vi "MGCC_FntStaMach_subMG_Identification.vi"(6 "Abnormal_enable_input":bool[][](array[boolean]), 7 "Abnormal input":string[](array[string]), 9 "Previous_states 2":string[](array[string]), 10 "Previous_node":i32[](array[numeric]), 11 "Turns":dbl) -> (0 "error out 2":errorcluster, 1 "Next_States":string[](array[string]), 3 "Next_node":dbl[](array[numeric]), 4 "Abnormal_enable_output":bool[][](array[boolean]), 5 "Abnormal_output":string[](array[string]))   [LabVIEW 2016]
uses:
  <vilib>/imath/engines/lvmath/Plug In/_Char/NIMS_CH_character datatype.ctl
  MGCC_FntStaMach_gobal.vi
  <vilib>/Utility/error.llb/Error Cluster From Error Code.vi
  <vilib>/imath/engines/lvmath/Plug In/_Char/NIMS_CH_String to Character Array.vi
  <vilib>/imath/engines/lvmath2/RunTimeEngine/RunTimeType/NIMS_RunTimeType_From StrictType (excl LVString).vi
  <instcachedir>/0/NIMS_RunTimeType_From StrictType (excl LVString)_BBF44FB49F834B71AF7A14CCEDF8BECD.lvgen/NIMS_RunTimeType_From StrictType (excl LVString)_BBF44FB49F834B71AF7A14CCEDF8BECD_006.vi
  <vilib>/imath/engines/lvmath2/RunTimeEngine/Struct/NIMS_StructSetField.vi
  <vilib>/imath/engines/lvmath2/RunTimeEngine/IndexRead/NIMS M(S,$).vi
  <instcachedir>/0/NIMS M(S,$)_F24F360562DE41D8BE234322A2E15C65.lvgen/NIMS M(S,$)_F24F360562DE41D8BE234322A2E15C65_000.vi
  <vilib>/imath/engines/lvmath2/RunTimeEngine/BuiltInFunctions/findnz/NIMS_[1o]_findnz(GRowV).vi
  <instcachedir>/0/NIMS_[1o]_findnz(GRowV)_1AF74843B4874134ADE908C0A4A72F3C.lvgen/NIMS_[1o]_findnz(GRowV)_1AF74843B4874134ADE908C0A4A72F3C_000.vi
  <vilib>/imathl/engines/lvmath/Functions/Error Handling/Create Error.vi
  <vilib>/imath/engines/lvmath2/RunTimeEngine/BuiltInFunctions/length/NIMS_length(GV).vi
  <instcachedir>/0/NIMS_length(GV)_08A3D13377FD4E4B96F5795FBF3698FA.lvgen/NIMS_length(GV)_08A3D13377FD4E4B96F5795FBF3698FA_000.vi
  <vilib>/imath/engines/lvmath2/RunTimeEngine/RangeToken/NIMS_Range_R3 - Integer.vi
  <instcachedir>/0/NIMS_Range_R3 - Integer_A435E2FF893B4C718FD5055FE39FE2F6.lvgen/NIMS_Range_R3 - Integer_A435E2FF893B4C718FD5055FE39FE2F6_000.vi
  <vilib>/imath/engines/lvmath2/RunTimeEngine/CommandStatement/MC_CommandStatement_break.vi
  <vilib>/imath/engines/lvmath2/RunTimeEngine/BuiltInFunctions/is_empty/NIMS_is_empty(GV).vi
  <instcachedir>/0/NIMS_is_empty(GV)_FC7E7C3D9544432CB6AA2416ADCF6D56.lvgen/NIMS_is_empty(GV)_FC7E7C3D9544432CB6AA2416ADCF6D56_000.vi
  <vilib>/imath/engines/lvmath2/RunTimeEngine/IndexRead/NIMS M($,S).vi
  <instcachedir>/0/NIMS M($,S)_3E5749BBB62E49528D4765A77F1F6D98.lvgen/NIMS M($,S)_3E5749BBB62E49528D4765A77F1F6D98_000.vi
  <vilib>/imath/engines/lvmath2/RunTimeEngine/RowToken/NIMS_RowToken_M_CV.vi
  <instcachedir>/0/NIMS_RowToken_M_CV_FA79F1D1D17D44459F3ED8E09EE8B625.lvgen/NIMS_RowToken_M_CV_FA79F1D1D17D44459F3ED8E09EE8B625_000.vi
  <vilib>/imath/engines/lvmath2/RunTimeEngine/ErrorHandling/NIMS_Create Error From Enums.vi
  <vilib>/imath/engines/lvmath2/RunTimeEngine/IndexRead/NIMS V(S).vi
  <instcachedir>/0/NIMS V(S)_0488751826AF41519A22953C041130DC.lvgen/NIMS V(S)_0488751826AF41519A22953C041130DC_000.vi
  <vilib>/imath/engines/lvmath2/RunTimeEngine/IndexRead/NIMS V(V).vi
  <instcachedir>/0/NIMS V(V)_298D9CB7BFEB42B8BC8D9C3C28AE8C70.lvgen/NIMS V(V)_298D9CB7BFEB42B8BC8D9C3C28AE8C70_002.vi
  <vilib>/imath/engines/lvmath2/RunTimeEngine/IndexReplace/NIMS V(S)=V.vi
  <instcachedir>/0/NIMS V(S)=V_623363232DF04CF88CEE4AC156064DF2.lvgen/NIMS V(S)=V_623363232DF04CF88CEE4AC156064DF2_003.vi
  <instcachedir>/0/NIMS_[1o]_findnz(GRowV)_1AF74843B4874134ADE908C0A4A72F3C.lvgen/NIMS_[1o]_findnz(GRowV)_1AF74843B4874134ADE908C0A4A72F3C_002.vi
  <vilib>/imath/engines/lvmath2/RunTimeEngine/VariableToken/NIMS_VariableToken_CondDefinedDefinedByReplace.vi
  <instcachedir>/0/NIMS_VariableToken_CondDefinedDefinedByReplace_D162CFFC24174562A9FEA619A91E1A56.lvgen/NIMS_VariableToken_CondDefinedDefinedByReplace_D162CFFC24174562A9FEA619A91E1A56_006.vi
  <vilib>/imath/engines/lvmath2/RunTimeEngine/IndexReplace/NIMS V(S)=S.vi
  <instcachedir>/0/NIMS V(S)=S_57E16554CB8B4B90AAB163894F717546.lvgen/NIMS V(S)=S_57E16554CB8B4B90AAB163894F717546_002.vi
  <vilib>/imath/engines/lvmath2/RunTimeEngine/BuiltInFunctions/size/NIMS_[I32,I32]=size(GM).vi
  <instcachedir>/0/NIMS_[I32,I32]=size(GM)_B0A6EC1255BB4C8AB801FE6F734128D9.lvgen/NIMS_[I32,I32]=size(GM)_B0A6EC1255BB4C8AB801FE6F734128D9_000.vi
  <vilib>/imath/engines/lvmath2/RunTimeEngine/Struct/NIMS_Struct_Cell Array To String Array.vi
  <vilib>/imath/engines/lvmath2/RunTimeEngine/IndexRead/NIMS V(R2).vi
  <instcachedir>/0/NIMS V(R2)_C76619605A0E4E9F8B2FA9389712AC47.lvgen/NIMS V(R2)_C76619605A0E4E9F8B2FA9389712AC47_002.vi
  <vilib>/imath/engines/lvmath2/RunTimeEngine/NodeEndStatement/NIMS_NodeEndStatement_Output.vi
  <instcachedir>/0/NIMS_NodeEndStatement_Output_53EC0D466D134D7ABD903AC30B43404B.lvgen/NIMS_NodeEndStatement_Output_53EC0D466D134D7ABD903AC30B43404B_004.vi
  <instcachedir>/0/NIMS_NodeEndStatement_Output_53EC0D466D134D7ABD903AC30B43404B.lvgen/NIMS_NodeEndStatement_Output_53EC0D466D134D7ABD903AC30B43404B_002.vi
  <instcachedir>/0/NIMS_NodeEndStatement_Output_53EC0D466D134D7ABD903AC30B43404B.lvgen/NIMS_NodeEndStatement_Output_53EC0D466D134D7ABD903AC30B43404B_031.vi
  <instcachedir>/0/NIMS_NodeEndStatement_Output_53EC0D466D134D7ABD903AC30B43404B.lvgen/NIMS_NodeEndStatement_Output_53EC0D466D134D7ABD903AC30B43404B_005.vi
  <vilib>/imath/engines/lvmath2/RunTimeEngine/ErrorHandling/NIMS_Finalize Error.vi
  <vilib>/ErrorRing/Error Ring.xnode
panel:
  out "emptyarray":i32[](array[numeric])
  out "temp_node":dbl[][](array[numeric])
  out "Next_states":string[](array[string])
  out "error out":errorcluster
  out "f_MGCC_OnliTopolden_node":dbl[][](array[numeric])
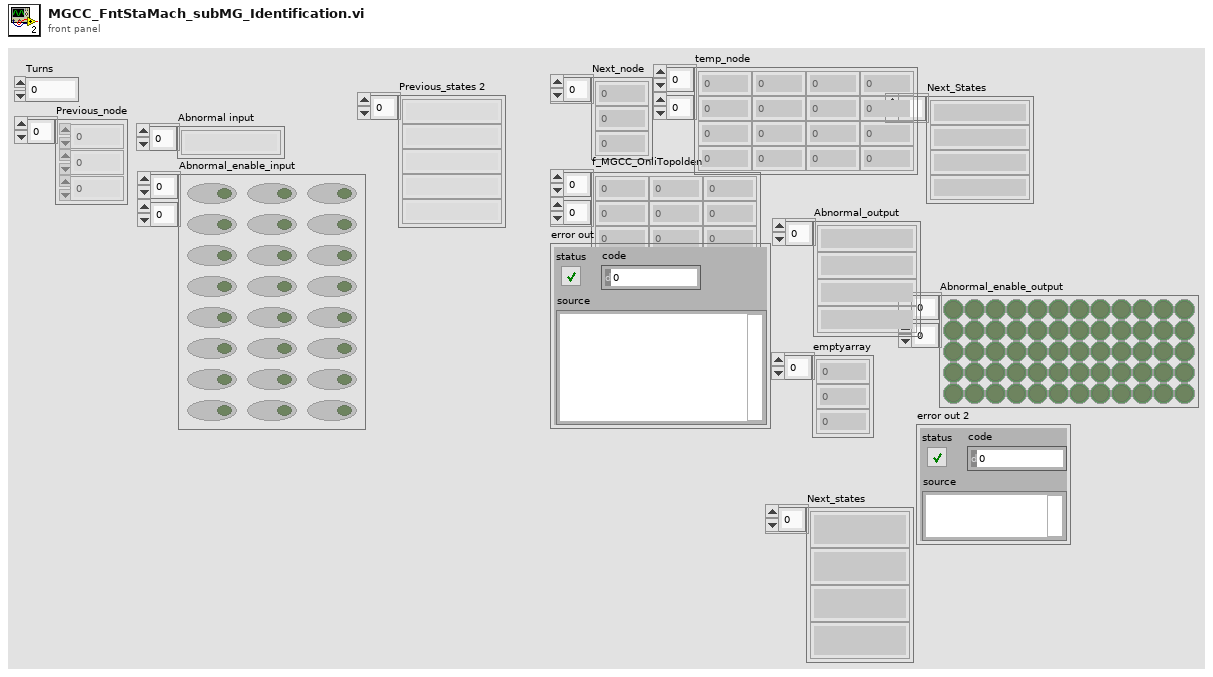
[diagram p1: front panel]
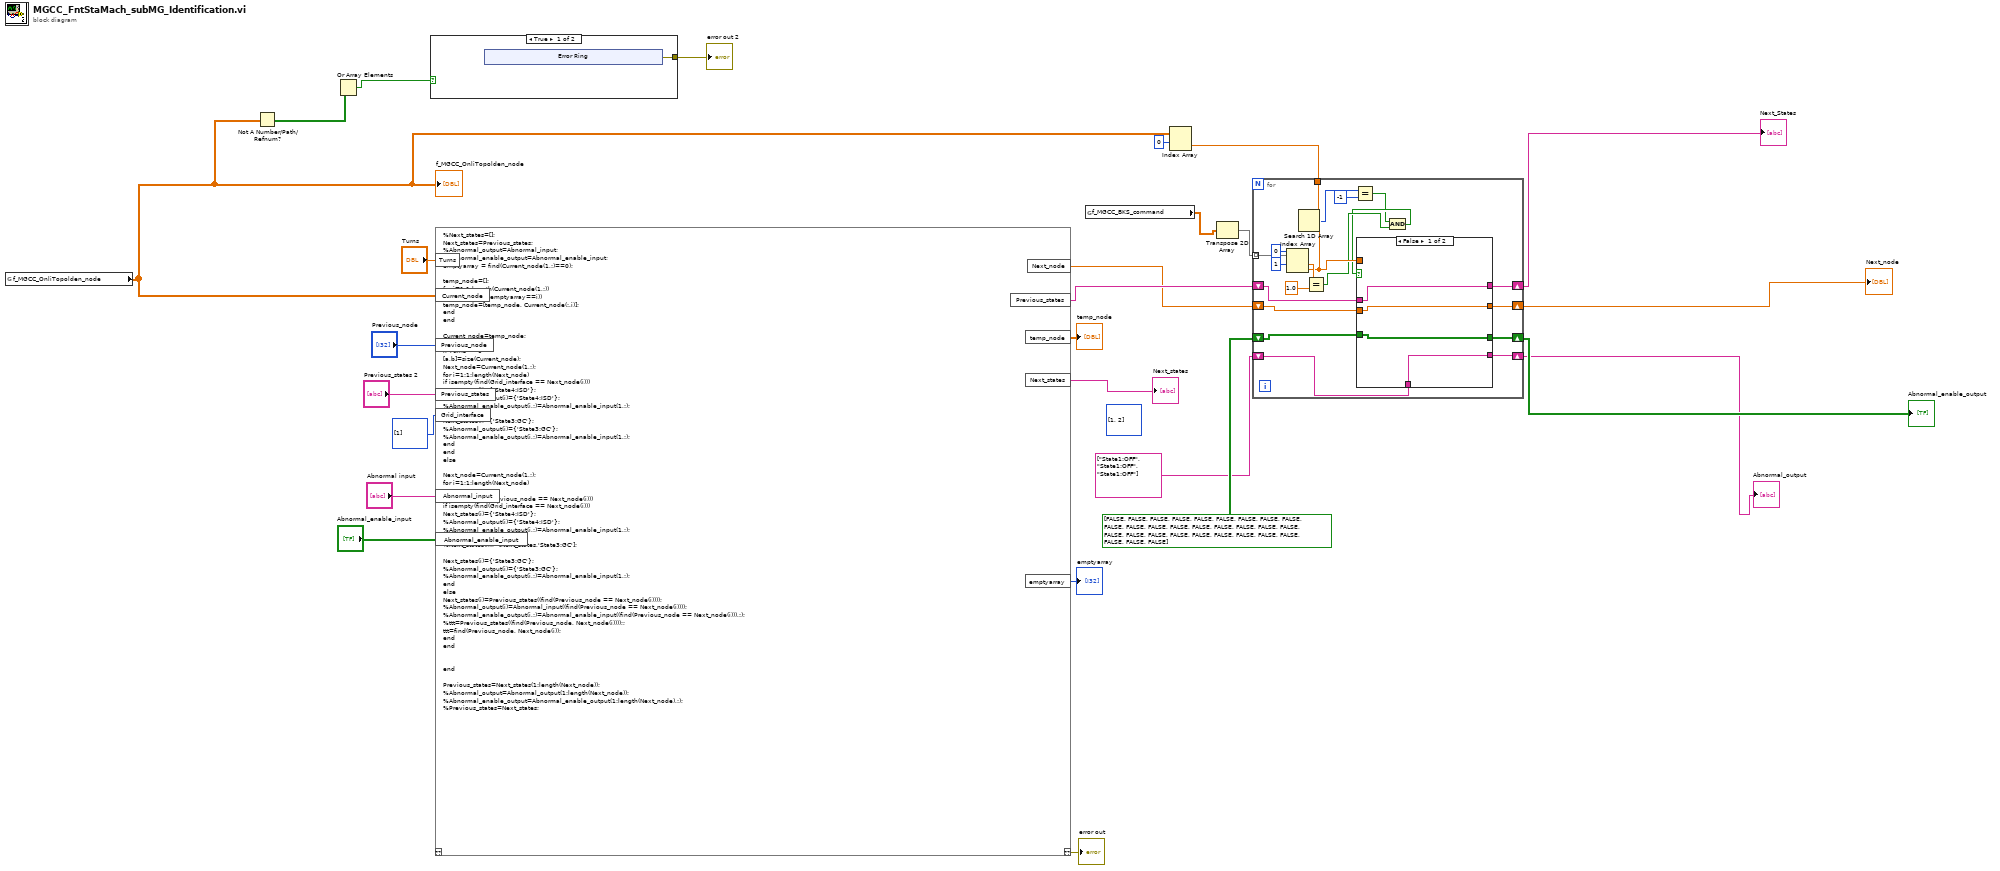
[diagram p0: block diagram]
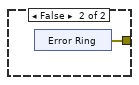
[diagram p2: hidden frame]
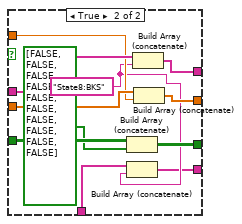
[diagram p3: hidden frame]
diagram:
  (unwired) i32[] [1, 2]
  n1 = global read "MGCC_FntStaMach_gobal.vi" "f_MGCC_OnliTopolden_node"() -> (w3:dbl[][])
  "f_MGCC_OnliTopolden_node" <- w3
  n2 = Not A Number/Path/Refnum?(number/path/refnum=w3) -> (NaN/Path/Refnum?=w8:bool[][])
  n3 = Or Array Elements(Boolean array=w8) -> (logical OR=w7:bool)
  n4 = case shown="True" w7 {
    tunnel: [w27 w33] -> w6
    frame True {
      n5 = xnode "Error Ring"() -> ("error out"=w27:errorcluster)
    }
    frame False {
      n6 = xnode "Error Ring"() -> ("error out"=w33:errorcluster)
    }
  }
  "error out 2" <- w6
  n7 = mathscript code="%Next_states=[];\nNext_states=Previous_states;\n%Abnormal_output=Abnormal_input;\n%Abnormal_enable_output=Abnormal_enable_input;\nemptyarray = find(Current_node(1,:)==0);\n\ntemp_node=[];\nfor i=1:1:length(Current_node(1,:))\nif isempty(find(emptyarray==i))\ntemp_node=[temp_node, Current_node(:,i)];\nend\nend\n\nCurrent_node=temp_node;\n\nif Turns ==0\n[a,b]=size(Current_node);\nNext_node=Current_node(1,:);\nfor i=1:1:length(Next_node)\nif isempty(find(Grid_interface == Next_node(i)))\nNext_states(i)={'State4:ISD'};\n%Abnormal_output(i)={'State4:ISD'};\n%Abnormal_enable_output(i,:)=Abnormal_enable_input(1,:);\nelse\nNext_states(i)={'State3:GC'};\n%Abnormal_output(i)={'State3:GC'};\n%Abnormal_enable_output(i,:)=Abnormal_enable_input(1,:);\nend\nend\nelse\n\nNext_node=Current_node(1,:);\nfor i=1:1:length(Next_node)\n\nif isempty(find(Previous_node == Next_node(i)))\nif isempty(find(Grid_interface == Next_node(i)))\nNext_states(i)={'State4:ISD'};\n%Abnormal_output(i)={'State4:ISD'};\n%Abnormal_enable_output(i,:)=Abnormal_enable_input(1,:);\nelse\n%Next_states(i,:)=[Next_states,'State3:GC'];\n\nNext_states(i)={'State3:GC'};\n%Abnormal_output(i)={'State3:GC'};\n%Abnormal_enable_output(i,:)=Abnormal_enable_input(1,:);\nend\nelse\nNext_states(i)=Previous_states((find(Previous_node == Next_node(i))));\n%Abnormal_output(i)=Abnormal_input((find(Previous_node == Next_node(i))));\n%Abnormal_enable_output(i,:)=Abnormal_enable_input((find(Previous_node == Next_node(i))),:);\n%ttt=Previous_states((find(Previous_node, Next_node(i))));;\nttt=find(Previous_node, Next_node(i));\nend\nend\n\n\nend\n\nPrevious_states=Next_states(1:length(Next_node));\n%Abnormal_output=Abnormal_output(1:length(Next_node));\n%Abnormal_enable_output=Abnormal_enable_output(1:length(Next_node),:);\n%Previous_states=Next_states;"("Current_node"=w3, "Turns"="Turns", "Previous_node"="Previous_node", "Previous_states"="Previous_states 2", "Grid_interface"=i32[] [1], "Abnormal_input"="Abnormal input", "Abnormal_enable_input"="Abnormal_enable_input") -> ("??"=→"error out":errorcluster, "Next_node"=w19:dbl[], "Previous_states"=w21:string[], "Next_states"=→"Next_states":string[], "temp_node"=→"temp_node":dbl[][], "emptyarray"=→"emptyarray":i32[])  [unwired: 1 in]
  n8 = global read "MGCC_FntStaMach_gobal.vi" "f_MGCC_BKS_command"() -> (w15:dbl[][])
  n9 = Index Array(array=w3, index (row)=0) -> (element=w12:dbl[])  [unwired: 1 in]
  n10 = Transpose 2D Array(2D array=w15) -> (transposed array=w14:dbl[][])
  n11 = for {
    tunnel: w14 -> [w54] mode=indexing
    shift-right: [w49] -> w20
    shift-left: w21 -> [w50]
    shift-right: [w46] -> w18
    shift-left: w19 -> [w48]
    shift-right: [w44] -> w17
    shift-left: bool[][] [[FALSE, FALSE, FALSE, FALSE, FALSE, FALSE, FALSE, FALSE, FALSE, FALSE], [FALSE, FALSE, FALSE, FALSE, FALSE, FALSE, FALSE, FALSE, FALSE, FALSE], [FALSE, FALSE, FALSE, FALSE, FALSE, FALSE, FALSE, FALSE, FALSE, FALSE]] ("ABN Function Enable output") -> [w45]
    shift-right: [w42] -> w16
    shift-left: string[] ["State1:OFF", "State1:OFF", "State1:OFF"] ("ABN State output") -> [w43]
    tunnel: w12 -> [w41]
    n12 = Index Array(array=w54, index #1=1 ("index"), index #2=0 ("index")) -> (element #1=w52:dbl, element #2=w40:dbl)
    n13 = Search 1D Array(1D array=w41, element=w40) -> (index of element=w37:i32)  [unwired: 1 in]
    n14 = Equal?(x=w52, y=1.0) -> (x = y?=w39:bool)
    n15 = Equal?(x=w37, y=-1) -> (x = y?=w35:bool)
    n16 = And(x=w35, y=w39) -> (x .and. y?=w38:bool)
    n17 = case shown="False" w38 {
      tunnel: w50 -> [w58 w69]
      tunnel: [w58 w68] -> w49
      tunnel: w48 -> [w57 w67]
      tunnel: w40 -> [_ w66]
      tunnel: [w57 w65] -> w46
      tunnel: w45 -> [w56 w64]
      tunnel: [w56 w62] -> w44
      tunnel: w43 -> [w55 w61]
      tunnel: [w55 w59] -> w42
      frame False {
      }
      frame True {
        w60 = "State8:BKS"
        n18 = Build Array (concatenate)(w64, bool[] [FALSE, FALSE, FALSE, FALSE, FALSE, FALSE, FALSE, FALSE, FALSE, FALSE]) -> (w62:bool[][])
        n19 = Build Array (concatenate)(w61, w60) -> (w59:string[])
        n20 = Build Array (concatenate)(w69, w60) -> (w68:string[])
        n21 = Build Array (concatenate)(w67, w66) -> (w65:dbl[])
      }
    }
  }
  "Next_node" <- w18
  "Next_States" <- w20
  "Abnormal_enable_output" <- w17
  "Abnormal_output" <- w16
